vi "OE1022D_RS232_Query Data.vi"(0 "VISA resource name":refnum<visa-resource-name>, 11 "Error in (no error)":errorcluster caption="error out（no error）") -> (4 "VISA resource  out":refnum<visa-resource-name>, 6 "Parameter Values":T1, 8 "Data Array":dbl[](array[numeric]), 10 "Output String":string, 15 "Error out":errorcluster caption="error out")   [LabVIEW 2011]
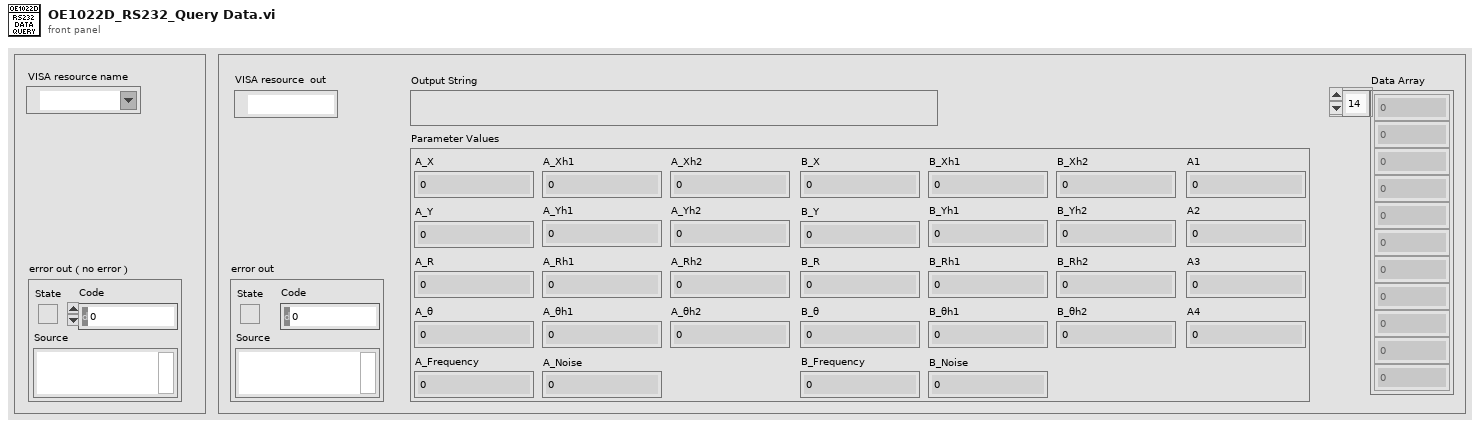
[diagram p1: front panel]
types:
  T1 = cluster{"A_X":dbl, "A_Y":dbl, "A_R":dbl, "A_θ":dbl, "A_Frequency":dbl, "A_Noise":dbl, "A_Xh1":dbl, "A_Yh1":dbl, "A_Rh1":dbl, "A_θh1":dbl, "A_Xh2":dbl, "A_Yh2":dbl, "A_Rh2":dbl, "A_θh2":dbl, "B_X":dbl, "B_Y":dbl, "B_R":dbl, "B_θ":dbl, "B_Frequency":dbl, "B_Noise":dbl, "B_Xh1":dbl, "B_Yh1":dbl, "B_Rh1":dbl, "B_θh1":dbl, "B_Xh2":dbl, "B_Yh2":dbl, "B_Rh2":dbl, "B_θh2":dbl, "A1":dbl, "A2":dbl, "A3":dbl, "A4":dbl}
  T2 = enum16{"ISRC", "IGND", "ICPL", "ILIN", "PHAS", "FMOD", "RSLP", "FREQ", "SWPT", "SLLM", "SULM", "SSLL", "SSLG", "STLM", "SWRM", "IRNG", "SENS", "RMOD", "OFLT", "OFSL", "SYNC", "DMOD", "HARM", "DARB", "SWVT", "SLVL", "SVLL", "SVUL", "SVSL", "SVSG", "SVTM", "SVRM", "RALL", "SNAP", "OUTP", "OAUX", "COUT", "CAUX", "COFP", "CEXP", "FPOP", "OEXP", "*IDN", "*RST", "OVLD", "INOV", "GNOV", "*PLL", "SSET", "RSET", "AGAN", "APHS", "ARSV", "ASCL", "EQCD", "EQCS", "SPED", "SRAT", "SLEN", "SSLE", "STRG", "SPRM", "STRD", "PAUS", "REST", "SPTS", "TRCA", "TEMP", "RSTU", "IHNZ", "DEQU", "SADD", "ARNG", "CSPE", "ISRCD", "IGNDD", "ICPLD", "ILIND", "PHASD", "FMODD", "RSLPD", "FREQD", "SWPTD", "SLLMD", "SULMD", "SSLLD", "SSLGD", "STLMD", "SWRMD", "SENSD", "RMODD", "OFLTD", "OFSLD", "SYNCD", "HARMD", "EQCDD", "EQCSD", "SNAPD", "OUTPD", "SWVTD", "SLVLD", "SVLLD", "SVULD", "SVSLD", "SVSGD", "SVTMD", "SVRMD", "SVDCD", "ARSVD", "AGAND", "APHSD", "ASCLD", "FPOPD", "CAUXD", "OEXPD", "SPEDD", "SRATD", "SLEND", "SSLED", "STRGD", "SPRMD", "STRDD", "PAUSD", "RESTD", "SPTSD", "TRCAD", "*IDND", "*RSTD", "INOVD", "GNOVD", "*PLLD", "SSETD", "RSETD", "RALLD"}
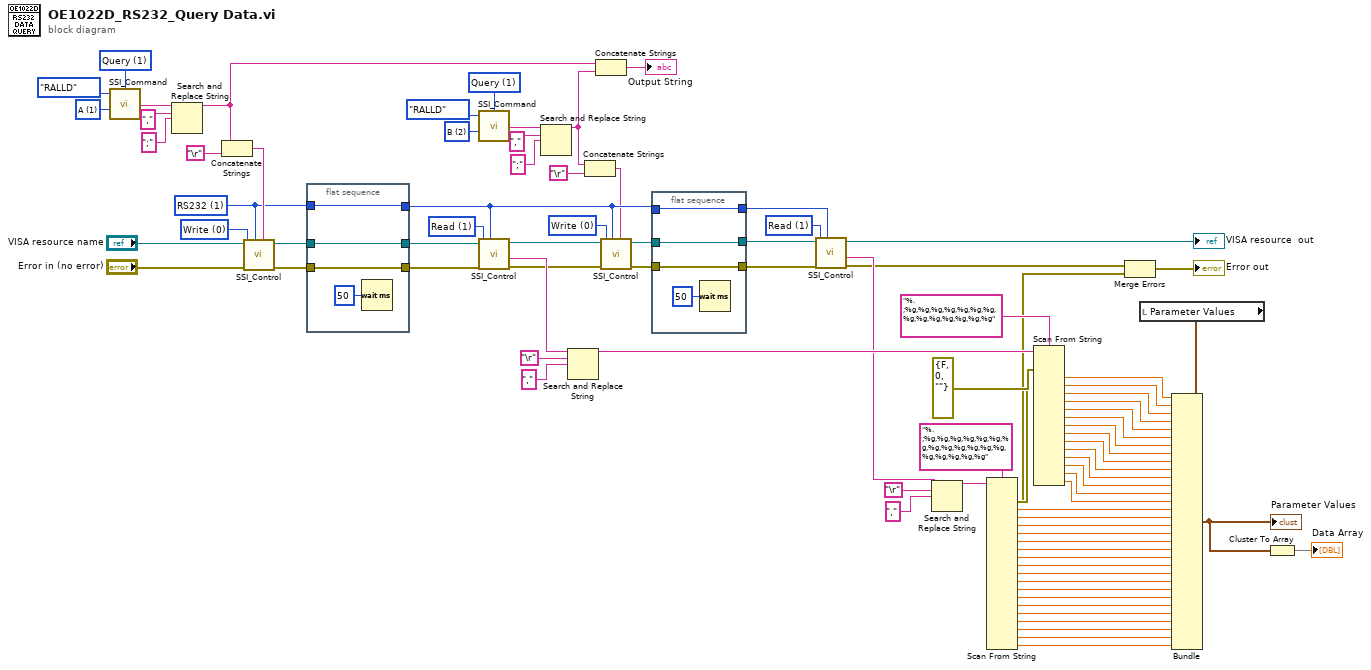
[diagram p0: block diagram]
diagram:
  w55 = u16 0 items=["Write", "Read"] ("Control")
  w60 = u16 1 items=["Write", "Read"] ("Control")
  w64 = u16 2 items=["A"=1, "B"=2] ("channel")
  w70 = u16 1 items=["A"=1, "B"=2] ("channel")
  w66 = u16 1 items=["Set", "Query"] ("Opera")
  w71 = u16 1 items=["Set", "Query"] ("Opera")
  w80 = u16 1 items=["USB", "RS232", "GPIB", "Ethernet"] ("Remote Mode")
  w82 = u16 1 items=["Write", "Read"] ("Control")
  w87 = u16 0 items=["Write", "Read"] ("Control")
  n1 = call "SSI_Command.vi"("Opera"=w66, "channel"=w70, "Command Type"=T2."RALLD") -> ("Output string"=w67:string)  [unwired: 1 in]
  n2 = Search and Replace String(input string=w67, search string="," ("搜索字符串"), replace string=";") -> (result string=w52:string)  [unwired: 5 in, 3 out]
  n3 = Concatenate Strings(w52, "\r") -> (w81:string)
  n4 = call "SSI_Control.vi"("Write Buffer"=w81, "Remote Mode"=w80, "Error in (no error)"="Error in (no error)", "Control"=w87, "VISA resource name"="VISA resource name") -> ("Error out"=w85:errorcluster, "VISA resource  out"=w86:refnum<visa-resource-name>)  [unwired: 3 in, 2 out]
  n5 = flat-sequence {
    tunnel: w86 -> [w93]
    tunnel: w85 -> [w92]
    tunnel: [w93] -> w84
    tunnel: [w92] -> w83
    tunnel: [w90] -> w56
    tunnel: w80 -> [w90]
    frame #0 {
      n6 = Wait (ms)(milliseconds to wait=u32 50 ("等待时间（毫秒）")) -> ()  [unwired: 1 out]
    }
  }
  n7 = call "SSI_Command.vi"("Opera"=w71, "channel"=w64, "Command Type"=T2."RALLD") -> ("Output string"=w78:string)  [unwired: 1 in]
  n8 = call "SSI_Control.vi"("Remote Mode"=w56, "Error in (no error)"=w83, "Control"=w82, "VISA resource name"=w84) -> ("Error out"=w62:errorcluster, "Read Buffer"=w74:string, "VISA resource  out"=w63:refnum<visa-resource-name>)  [unwired: 4 in, 1 out]
  n9 = Search and Replace String(input string=w78, search string="," ("搜索字符串"), replace string=";") -> (result string=w51:string)  [unwired: 5 in, 3 out]
  n10 = Search and Replace String(input string=w74, search string="\r", replace string=",") -> (result string=w14:string)  [unwired: 5 in, 3 out]
  n11 = Concatenate Strings(w51, "\r") -> (w53:string)
  n12 = Concatenate Strings(w52, w51) -> (→"Output String":string)
  n13 = call "SSI_Control.vi"("Write Buffer"=w53, "Remote Mode"=w56, "Error in (no error)"=w62, "Control"=w55, "VISA resource name"=w63) -> ("Error out"=w7:errorcluster, "VISA resource  out"=w61:refnum<visa-resource-name>)  [unwired: 3 in, 2 out]
  n14 = flat-sequence {
    tunnel: [w97] -> w59
    tunnel: w61 -> [w97]
    tunnel: w56 -> [w96]
    tunnel: [w96] -> w57
    tunnel: w7 -> [w94]
    tunnel: [w94] -> w6
    frame #0 {
      n15 = Wait (ms)(milliseconds to wait=u32 50 ("等待时间（毫秒）")) -> ()  [unwired: 1 out]
    }
  }
  n16 = call "SSI_Control.vi"("Remote Mode"=w57, "Error in (no error)"=w6, "Control"=w60, "VISA resource name"=w59) -> ("Error out"=w5:errorcluster, "Read Buffer"=w9:string, "VISA resource  out"=→"VISA resource  out":refnum<visa-resource-name>)  [unwired: 4 in, 1 out]
  n17 = Search and Replace String(input string=w9, search string="\r", replace string=",") -> (result string=w8:string)  [unwired: 5 in, 3 out]
  n18 = Scan From String(format string="%.;%g,%g,%g,%g,%g,%g,%g,%g,%g,%g,%g,%g,%g,%g" ("格式字符串"), input string=w14, error in=errorcluster {"status"=FALSE, "code"=0, "source"=""} ("error constant")) -> (error out=w2:errorcluster, output 1=w18:dbl, output 2=w17:dbl, output 3=w19:dbl, output 4=w20:dbl, output 5=w21:dbl, output 6=w22:dbl, output 7=w23:dbl, output 8=w24:dbl, output 9=w25:dbl, output 10=w26:dbl, output 11=w27:dbl, output 12=w28:dbl, output 13=w29:dbl, output 14=w30:dbl)  [unwired: 15 in, 2 out]
  n19 = Scan From String(format string="%.;%g,%g,%g,%g,%g,%g,%g,%g,%g,%g,%g,%g,%g,%g,%g,%g,%g,%g" ("格式字符串"), input string=w8, error in=w2) -> (error out=w1:errorcluster, output 1=w32:dbl, output 2=w33:dbl, output 3=w34:dbl, output 4=w35:dbl, output 5=w36:dbl, output 6=w37:dbl, output 7=w38:dbl, output 8=w39:dbl, output 9=w40:dbl, output 10=w41:dbl, output 11=w42:dbl, output 12=w43:dbl, output 13=w44:dbl, output 14=w45:dbl, output 15=w46:dbl, output 16=w47:dbl, output 17=w48:dbl, output 18=w49:dbl)  [unwired: 19 in, 2 out]
  n20 = Merge Errors(w5, w1) -> (→"Error out":errorcluster)
  n21 = local read "Parameter Values"() -> (w15:T1)
  n22 = Bundle(cluster=w15, "A_X"=w18, "A_Y"=w17, "A_R"=w19, "A_θ"=w20, "A_Frequency"=w21, "A_Noise"=w22, "A_Xh1"=w23, "A_Yh1"=w24, "A_Rh1"=w25, "A_θh1"=w26, "A_Xh2"=w27, "A_Yh2"=w28, "A_Rh2"=w29, "A_θh2"=w30, "B_X"=w32, "B_Y"=w33, "B_R"=w34, "B_θ"=w35, "B_Frequency"=w36, "B_Noise"=w37, "B_Xh1"=w38, "B_Yh1"=w39, "B_Rh1"=w40, "B_θh1"=w41, "B_Xh2"=w42, "B_Yh2"=w43, "B_Rh2"=w44, "B_θh2"=w45, "A1"=w46, "A2"=w47, "A3"=w48, "A4"=w49) -> (w16:T1)
  "Parameter Values" <- w16
  n23 = Cluster To Array(cluster=w16) -> (array=→"Data Array":dbl[])
